vi "USB Reset Device.vi"(11 "DevHandle":i32) -> (3 "function return":bool)   [LabVIEW 2010, in "usb_device.lvlib"]
doc: "bool WINAPI USB_ResetDevice(int DevHandle);"
uses:
  usb_device.lvlib
  USB2XXX/trunk/USB2XXX/USB2XXX/vs2010/Release/USB2XXX.dll
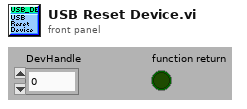
[diagram p1: front panel]
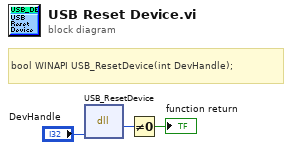
[diagram p0: block diagram]
diagram:
  # "bool WINAPI USB_ResetDevice(int DevHandle);"
  n1 = dll-call lib="E:/Projects/USB2XXX/trunk/USB2XXX/USB2XXX/vs2010/Release/USB2XXX.*" fn="USB_ResetDevice"("DevHandle"="DevHandle") -> (w2:u8)  [unwired: 4 in, 2 out]
  n2 = Not Equal To 0?(x=w2) -> (x != 0?=→"function return":bool)
